vi "Read LM Read Rate.vi"(8 "error in (no error)":errorcluster, 11 "Level Meter in":refnum<class "Level Meter.lvclass">) -> (0 "error out":errorcluster, 2 "fast?":bool caption="Fast Rate", 3 "Level Meter out":refnum<class "Level Meter.lvclass">)   [LabVIEW 2023, in "Level Meter.lvclass"]
uses:
  Level Meter.lvclass
  Level Meter.lvclass/Level Meter.ctl
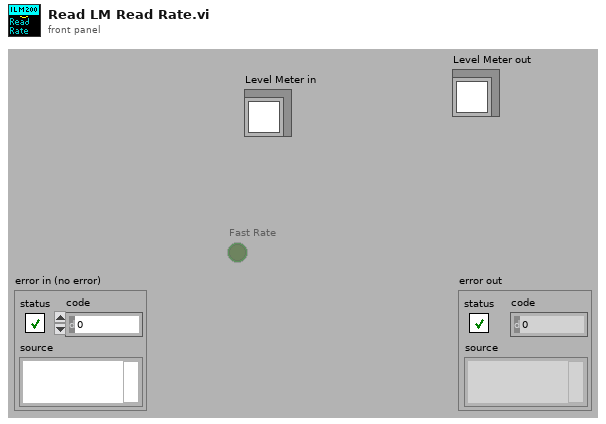
[diagram p1: front panel]
types:
  T1 = typedef "OxfordAddress.ctl" = cluster{"Com Port":i32, "ISOBUS Address":i32, "GPIB Address":i16, "Communication":enum16{"RS232", "ISOBUS", "GPIB", "Gateway"}}
  T2 = typedef "ILMChannelStatus.ctl" = cluster{"Probe current":bool, "Probe fast":bool, "Probe slow":bool, "Auto-fill":enum16{"End fill", "Not filling", "Filling", "Start filling"}, "Fill":bool, "Low level":bool, "Alm requested":bool, "Pre-pulse I":bool}
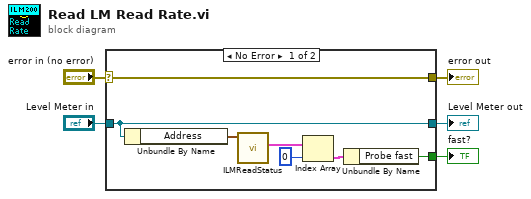
[diagram p0: block diagram]
diagram:
  n1 = case shown="No Error" "error in (no error)" {
    selector: "error in (no error)" -> [w7 w14]
    tunnel: [w8 _] -> w5
    tunnel: [w7 w14] -> w3
    tunnel: "Level Meter in" -> [w6 w13]
    tunnel: [w6 w13] -> w1
    frame No Error {
      n2 = Unbundle By Name(w6) -> ("Address"=w12:T1)
      n3 = call "ILMReadStatus.vi"("Instrument address"=w12) -> ("Channel"=w11:T2[])  [unwired: 2 in, 4 out]
      n4 = Index Array(array=w11, index=0) -> (element=w9:T2)
      n5 = Unbundle By Name(w9) -> ("Probe fast"=w8:bool)
    }
    frame Error {
    }
  }
  "fast?" <- w5
  "error out" <- w3
  "Level Meter out" <- w1
